vi "Read Timeout Iteration.vi"(8 "error in (no error)":errorcluster, 11 "LargeScrollbar in":refnum<class "LargeScrollbar.lvclass">) -> (0 "error out":errorcluster, 2 "Timeout Iteration":u32, 3 "LargeScrollbar out":refnum<class "LargeScrollbar.lvclass">)   [LabVIEW 2015, in "LargeScrollbar.lvclass"]
doc: "<b> </b> <b> </b>\n©2016 Q Software Innovations, LLC (QSI)\nwritten by Quentin Alldredge\nproduced in LabVIEW 2015\n\nsupport@qsoftwareinnovations.com\nwww.qsoftwareinnovations.com\n\nAll rights reserved.\n\nRedistribution and use in source and binary forms, with or without modification, are permitted provided that the following conditions are met:\n\n * Redistributions of source code must retain the above copyright notice, this list of conditions and the following disclaimer.\n * Redistributions in binary form must reproduce the above copyright notice, this list of conditions and the following disclaimer in the documentation and/or other materials provided with the distribution.\n * Neither the name of Q Software Innovations, LLC. nor the names of its contributors may be used to endorse or promote products derived from this software without specific prior written permission.\n\nTHIS SOFTWARE IS PROVIDED BY THE COPYRIGHT HOLDERS AND CONTRIBUTORS \"AS IS\" AND ANY EXPRESS OR IMPLIED WARRANTIES, INCLUDING, BUT NOT LIMITED TO, THE IMPLIED WARRANTIES OF MERCHANTABILITY AND FITNESS FOR A PARTICULAR PURPOSE ARE DISCLAIMED. IN NO EVENT SHALL THE COPYRIGHT OWNER OR CONTRIBUTORS BE LIABLE FOR ANY DIRECT, INDIRECT, INCIDENTAL, SPECIAL, EXEMPLARY, OR CONSEQUENTIAL DAMAGES (INCLUDING, BUT NOT LIMITED TO, PROCUREMENT OF SUBSTITUTE GOODS OR SERVICES; LOSS OF USE, DATA, OR PROFITS; OR BUSINESS INTERRUPTION) HOWEVER CAUSED AND ON ANY THEORY OF LIABILITY, WHETHER IN CONTRACT, STRICT LIABILITY, OR TORT (INCLUDING NEGLIGENCE OR OTHERWISE) ARISING IN ANY WAY OUT OF THE USE OF THIS SOFTWARE, EVEN IF ADVISED OF THE POSSIBILITY OF SUCH DAMAGE."
uses:
  LargeScrollbar.lvclass
  LargeScrollbar.lvclass/LargeScrollbar.ctl
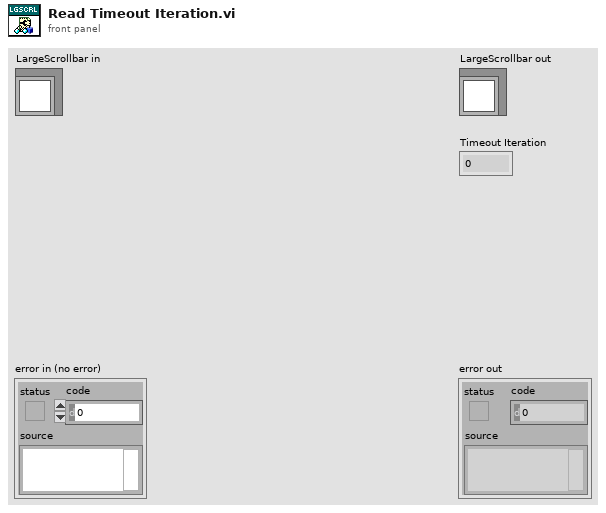
[diagram p1: front panel]
types:
  T1 = typedef "LargeScrollbar.lvclass/State Data.ctl" = cluster{"Direction":T2, "Timeout Iteration":u32}
  T2 = typedef "LargeScrollbar.lvclass/Direction.ctl" = enum16{"Decrement", "Increment"}
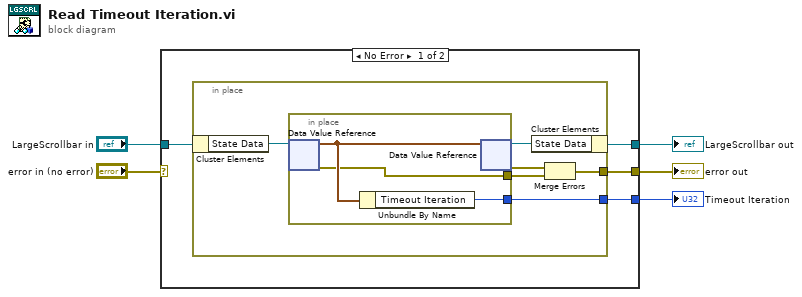
[diagram p0: block diagram]
diagram:
  n1 = case shown="No Error" "error in (no error)" {
    selector: "error in (no error)" -> [_ w20]
    tunnel: [w6 w20] -> w4
    tunnel: [w8 w19] -> w2
    tunnel: "LargeScrollbar in" -> [w9 w19]
    tunnel: [w7 _] -> w1
    frame No Error {
      n2 = in-place {
        in-place-border: [w14] -> w7
        in-place-border: [w11] -> w6
        n3 = in-place-cluster #1(w9) -> ("State Data"=w15:refnum<data-value>)
        n4 = in-place {
          in-place-border: [w17] -> w14
          in-place-border: [w16] -> w13
          n5 = in-place-dvr #2(w15) -> (w18:T1, w16:errorcluster)
          n6 = Unbundle By Name(w18) -> ("Timeout Iteration"=w17:u32)
          n7 = in-place-dvr #2(w18) -> (w10:refnum<data-value>, w12:errorcluster)
        }
        n8 = in-place-cluster #1("State Data"=w10) -> (w8:refnum<class "LargeScrollbar.lvclass">)
        n9 = Merge Errors(w12, w13) -> (w11:errorcluster)
      }
    }
    frame Error {
    }
  }
  "error out" <- w4
  "LargeScrollbar out" <- w2
  "Timeout Iteration" <- w1
